vi "Export_Waveforms_To_spreadsheet_File_1D.vi"(4 "header? (write header:T)":bool=TRUE, 5 "delimiter (Tab)":string="\t", 6 "append to file? (new file:F)":bool, 7 "prompt":string="Choose file to write.", 8 "error in (no error)":errorcluster, 9 "multiple time columns? (single:F)":bool, 10 "waveforms":waveform(dbl)[](array[waveform]), 11 "file path (dialog if empty)":path) -> (0 "error out":errorcluster, 3 "new file path (Not A Path if cancelled)":path)   [LabVIEW 2011]
doc: "Converts a waveform to a text string and writes the string to a new byte stream file or appends the string to an existing file. Wire data to the <B>Waveform</B> input to determine the polymorphic instance to use or manually select the instance."
panel:
  out "Array":string[](array[string])
  out "spreadsheet string":string
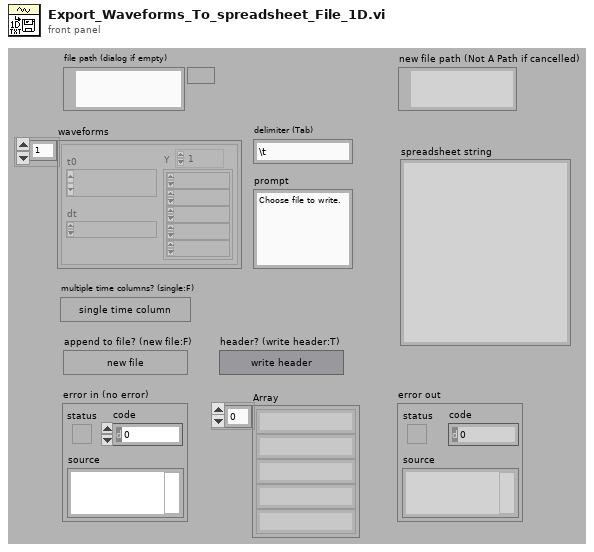
[diagram p1: front panel]
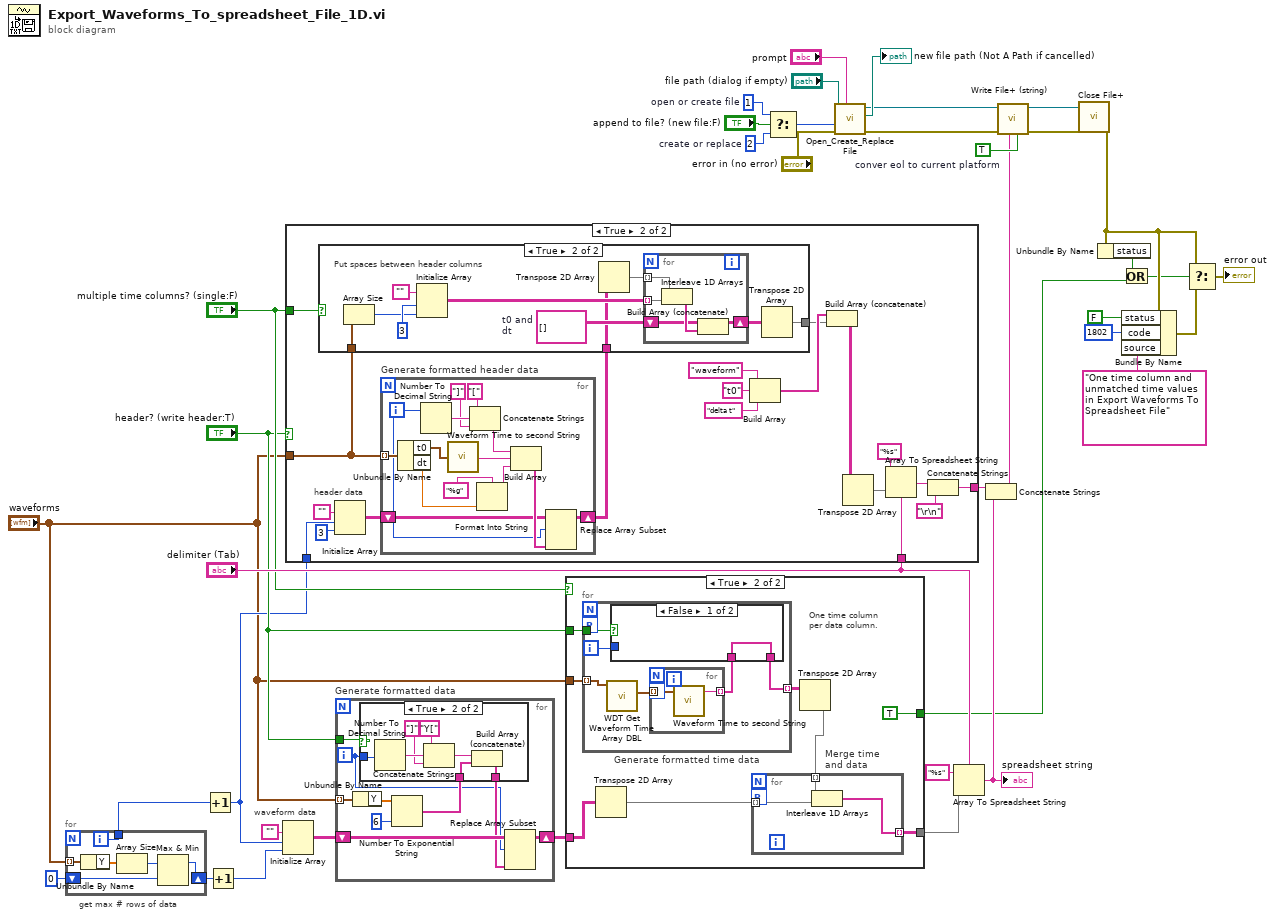
[diagram p0: block diagram]
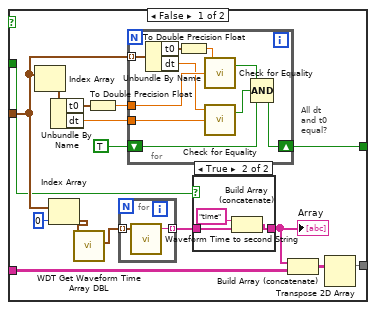
[diagram p2: hidden frame]
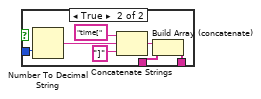
[diagram p4: hidden frame]
diagram:
  w31 = i16 2  # create or replace
  w33 = TRUE  # conver eol to current platform
  w38 = i16 1  # open or create file
  # "waveform data"
  # "get max # rows of data"
  n1 = for {
    tunnel: "waveforms" -> [w45] mode=indexing
    shift-right: [w41] -> w6
    shift-left: 0 -> [w42]
    tunnel: [w40] -> w4
    i -> [w40]
    n2 = Unbundle By Name(w45) -> ("Y"=w44:dbl[])
    n3 = Array Size(array=w44) -> (size(s)=w43:i32)
    n4 = Max & Min(x=w43, y=w42) -> (max(x,y)=w41:i32)  [unwired: 1 out]
  }
  n5 = Increment(x=w4) -> (x+1=w3:i32)
  n6 = Increment(x=w6) -> (x+1=w2:i32)
  n7 = Initialize Array("", w3, w2) -> (w5:string[][])
  n8 = case shown="True" "header? (write header:T)" {
    tunnel: "delimiter (Tab)" -> [_ w62]
    tunnel: "waveforms" -> [_ w56]
    tunnel: [_ w57] -> w22
    tunnel: "multiple time columns? (single:F)" -> [_ w54]
    tunnel: w3 -> [_ w47]
    frame False {
    }
    frame True {
      # "header data"
      n9 = Initialize Array("", w47, 3 ("dimension size")) -> (w46:string[][])
      n10 = for "Generate formatted header data" {
        tunnel: w56 -> [w87] mode=indexing
        shift-right: [w82] -> w52
        shift-left: w46 -> [w83]
        i -> [w81]
        n11 = Unbundle By Name(w87) -> ("t0"=w85:timestamp, "dt"=w92:dbl)
        n12 = Number To Decimal String(number=w81) -> (decimal integer string=w90:string)  [unwired: 1 in]
        n13 = call "Waveform Time to second String.vi"("t0"=w85) -> ("String"=w93:string)
        n14 = Concatenate Strings("[", w90, "]") -> (w91:string)
        n15 = Format Into String(format string="%g" ("Format String"), w92) -> (resulting string=w94:string)  [unwired: 2 in, 1 out]
        n16 = Build Array(w91, w93, w94) -> (w84:string[])
        n17 = Replace Array Subset(array=w83, new element=w84, index (row)=w81) -> (w82:string[][])  [unwired: 1 in]
      }
      n18 = case shown="True" w54 {
        tunnel: w56 -> [_ w75]
        tunnel: [w65 w70] -> w53
        tunnel: w52 -> [w65 w69]
        frame False {
          # "Leave the header data alone"
        }
        frame True {
          w73 = string[][] []  # t0 and dt
          # "Put spaces between header columns"
          n19 = Array Size(array=w75) -> (size(s)=w66:i32)
          n20 = Initialize Array("", 3 ("Dimension Size"), w66) -> (w72:string[][])
          n21 = Transpose 2D Array(2D array=w69) -> (transposed array=w68:string[][])
          n22 = for {
            shift-right: [w77] -> w71
            shift-left: w73 -> [w78]
            tunnel: w72 -> [w80] mode=indexing
            tunnel: w68 -> [w76] mode=indexing
            n23 = Interleave 1D Arrays(w76, w80) -> (w79:string[])
            n24 = Build Array (concatenate)(w78, w79) -> (w77:string[][])
          }
          n25 = Transpose 2D Array(2D array=w71) -> (transposed array=w70:string[][])
        }
      }
      n26 = Build Array("waveform", "t0", "delta t") -> (w55:string[])
      n27 = Build Array (concatenate)(w55, w53) -> (w50:string[][])
      n28 = Transpose 2D Array(2D array=w50) -> (transposed array=w51:string[][])
      n29 = Array To Spreadsheet String(delimiter (Tab)=w62, array=w51, 3:"%s" ("format string")) -> (spreadsheet string=w59:string)
      n30 = Concatenate Strings(w59, "\r\n") -> (w57:string)
    }
  }
  n31 = for "Generate formatted data" {
    tunnel: "waveforms" -> [w101] mode=indexing
    tunnel: "header? (write header:T)" -> [w98]
    shift-right: [w99] -> w21
    shift-left: w5 -> [w100]
    i -> [w95]
    n32 = Unbundle By Name(w101) -> ("Y"=w103:dbl[])
    n33 = Number To Exponential String(number=w103, precision (6)=i16 6) -> (E-format string=w97:string[])  [unwired: 2 in]
    n34 = case shown="True" w98 {
      tunnel: w95 -> [_ w108]
      tunnel: w97 -> [w104 w106]
      tunnel: [w104 w105] -> w96
      frame False {
      }
      frame True {
        n35 = Number To Decimal String(number=w108) -> (decimal integer string=w111:string)  [unwired: 1 in]
        n36 = Concatenate Strings("Y[", w111, "]") -> (w107:string)
        n37 = Build Array (concatenate)(w107, w106) -> (w105:string[])
      }
    }
    n38 = Replace Array Subset(array=w100, new element=w96, index (row)=w95) -> (w99:string[][])  [unwired: 1 in]
  }
  n39 = case shown="True" "multiple time columns? (single:F)" {
    tunnel: "waveforms" -> [w118 w151]
    tunnel: w21 -> [w125 w149]
    tunnel: [w123 w144] -> w20
    tunnel: [w117 TRUE] -> w10
    tunnel: "header? (write header:T)" -> [w114 w145]
    frame False {
      # "One time column - check for equal dt and t0"
      # "All dt\nand t0\nequal?"
      n40 = Index Array(array=w118) -> (element=w122:waveform(dbl))  [unwired: 1 in]
      n41 = Index Array(array=w118, index=0 ("Index")) -> (element=w113:waveform(dbl))
      n42 = Unbundle By Name(w122) -> ("t0"=w116:timestamp, "dt"=w119:dbl)
      n43 = call "WDT Get Waveform Time Array DBL.vi"("waveform in"=w113) -> ("X array"=w112:timestamp[])  [unwired: 9 in, 1 out]
      n44 = To Double Precision Float(number=w116) -> (double precision float=w120:dbl)
      n45 = for {
        tunnel: w112 -> [w142] mode=indexing
        tunnel: [w143] -> w126 mode=indexing
        n46 = call "Waveform Time to second String.vi"("t0"=w142) -> ("String"=w143:string)
      }
      n47 = for {
        tunnel: w118 -> [w141] mode=indexing
        shift-right: [w136] -> w117
        shift-left: TRUE -> [w135]
        tunnel: w120 -> [w139]
        tunnel: w119 -> [w137]
        n48 = Unbundle By Name(w141) -> ("t0"=w132:timestamp, "dt"=w138:dbl)
        n49 = To Double Precision Float(number=w132) -> (double precision float=w140:dbl)
        n50 = call <vilib>:"Check for Equality.vi"("n2"=w139, "n1"=w140) -> ("equal?"=w133:bool)  [unwired: 1 in, 1 out]
        n51 = call <vilib>:"Check for Equality.vi"("n2"=w137, "n1"=w138) -> ("equal?"=w134:bool)  [unwired: 1 in, 1 out]
        n52 = Compound Arithmetic op=AND(w133, w134, w135) -> (w136:bool)
      }
      n53 = case shown="True" w114 {
        tunnel: w126 -> [w128 w131]
        tunnel: [w128 w130] -> w115
        frame False {
        }
        frame True {
          n54 = Build Array (concatenate)("time", w131) -> (w130:string[])
        }
      }
      "Array" <- w115
      n55 = Build Array (concatenate)(w115, w125) -> (w124:string[][])
      n56 = Transpose 2D Array(2D array=w124) -> (transposed array=w123:string[][])
    }
    frame True {
      # "One time column\nper data column."
      n57 = for "Generate formatted time data" {
        tunnel: [w157] -> w150 mode=indexing
        tunnel: w151 -> [w156] mode=indexing
        tunnel: w145 -> [w159]
        workers-P: _ -> [_]
        i -> [w160]
        n58 = call "WDT Get Waveform Time Array DBL.vi"("waveform in"=w156) -> ("X array"=w155:timestamp[])  [unwired: 9 in, 1 out]
        n59 = for {
          tunnel: w155 -> [w169] mode=indexing
          tunnel: [w170] -> w158 mode=indexing
          workers-P: _ -> [_]
          n60 = call "Waveform Time to second String.vi"("t0"=w169) -> ("String"=w170:string)
        }
        n61 = case shown="False" w159 {
          tunnel: w160 -> [_ w165]
          tunnel: w158 -> [w161 w163]
          tunnel: [w161 w162] -> w157
          frame False {
          }
          frame True {
            n62 = Number To Decimal String(number=w165) -> (decimal integer string=w168:string)  [unwired: 1 in]
            n63 = Concatenate Strings("time[", w168, "]") -> (w164:string)
            n64 = Build Array (concatenate)(w164, w163) -> (w162:string[])
          }
        }
      }
      n65 = Transpose 2D Array(2D array=w149) -> (transposed array=w148:string[][])
      n66 = Transpose 2D Array(2D array=w150) -> (transposed array=w147:string[][])
      n67 = for "Merge time\nand data" {
        tunnel: w148 -> [w154] mode=indexing
        tunnel: w147 -> [w153] mode=indexing
        tunnel: [w152] -> w144 mode=indexing
        workers-P: _ -> [_]
        n68 = Interleave 1D Arrays(w153, w154) -> (w152:string[])
      }
    }
  }
  n69 = Select ("function")(t=w38, s="append to file? (new file:F)", f=w31) -> (s? t:f=w36:i16)
  n70 = call <vilib>:"Open_Create_Replace File.vi"("prompt"="prompt", "error in (no error)"="error in (no error)", "function (open:0)"=w36, "file path"="file path (dialog if empty)") -> ("error out"=w26:errorcluster, "new file path"=→"new file path (Not A Path if cancelled)":path, "refnum"=w25:refnum<file>)  [unwired: 4 in, 1 out]
  n71 = Array To Spreadsheet String(delimiter (Tab)="delimiter (Tab)", array=w20, 3:"%s" ("format (%.3f)")) -> (spreadsheet string=w24:string)
  "spreadsheet string" <- w24
  n72 = Concatenate Strings(w22, w24) -> (w23:string)
  n73 = call <vilib>:"Write File+ (string).vi"("convert eol? (no:F)"=w33, "string"=w23, "error in (no error)"=w26, "refnum"=w25) -> ("error out"=w37:errorcluster, "dup refnum"=w34:refnum<file>)  [unwired: 3 in, 1 out]
  n74 = call <vilib>:"Close File+.vi"("error in (no error)"=w37, "refnum"=w34) -> ("error out"=w17:errorcluster)  [unwired: 3 in, 2 out]
  n75 = Unbundle By Name(w17) -> ("status"=w16:bool)
  n76 = Or(x=w16, y=w10) -> (x .or. y?=w15:bool)
  n77 = Bundle By Name(cluster=w17, "status"=FALSE, "code"=1802, "source"="One time column and unmatched time values in Export Waveforms To Spreadsheet File") -> (w18:errorcluster)
  n78 = Select(t=w17, s=w15, f=w18) -> (s? t:f=→"error out":errorcluster)
